vi "19052_read_UT_status.vi"(8 "error in (no error)":errorcluster, 10 "timeout [s]":dbl=10.0 format="%0.2f", 11 "task/channels in":refnum<k21>) -> (0 "error out":errorcluster, 1 "Under  Test":bool, 3 "task out":refnum<k21>)   [LabVIEW 2015]
uses:
  <vilib>/DAQmx/read.llb/DAQmx Read (Digital 1D Bool 1Chan 1Samp).vi
  <vilib>/DAQmx/miscellaneous.llb/DAQmx Fill In Error Info.vi
panel:
  # "Read CHROMA 19052 UNDER TEST LED status"
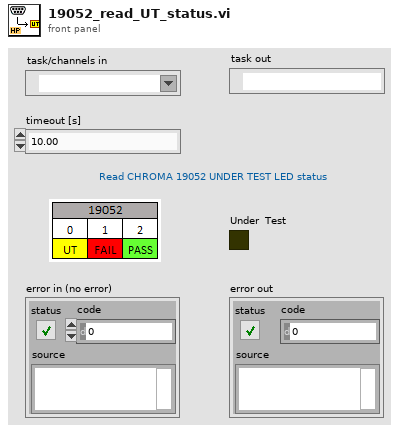
[diagram p1: front panel]
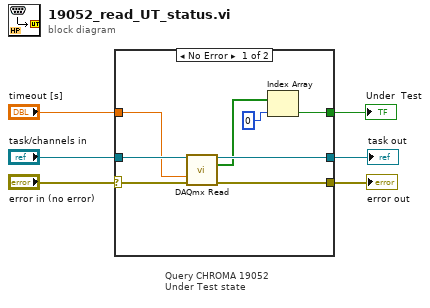
[diagram p0: block diagram]
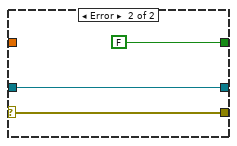
[diagram p2: hidden frame]
diagram:
  # "Query CHROMA 19052\nUnder Test state"
  n1 = case shown="No Error" "error in (no error)" {
    selector: "error in (no error)" -> [w9 w16]
    tunnel: [w14 FALSE ("Boolean")] -> w6
    tunnel: [w13 w16] -> w5
    tunnel: [w11 w17] -> w4
    tunnel: "task/channels in" -> [w10 w17]
    tunnel: "timeout [s]" -> [w8 _]
    frame No Error {
      n2 = call-poly <vilib>:"DAQmx Read.vi"("task/channels in"=w10, "timeout"=w8, "error in"=w9) -> ("task out"=w11:refnum<k21>, "data"=w7:bool[], "error out"=w13:errorcluster)  [unwired: 10 in]
      n3 = Index Array(array=w7, index=0) -> (element=w14:bool)
    }
    frame Error {
    }
  }
  "Under  Test" <- w6
  "error out" <- w5
  "task out" <- w4
